vi "delete_document.vi"(11 "did":string) -> ()   [LabVIEW 2019]
panel:
  out "Device Out":T1
  in  "Device In":T1
  out "error out":errorcluster
  in  "error in":errorcluster
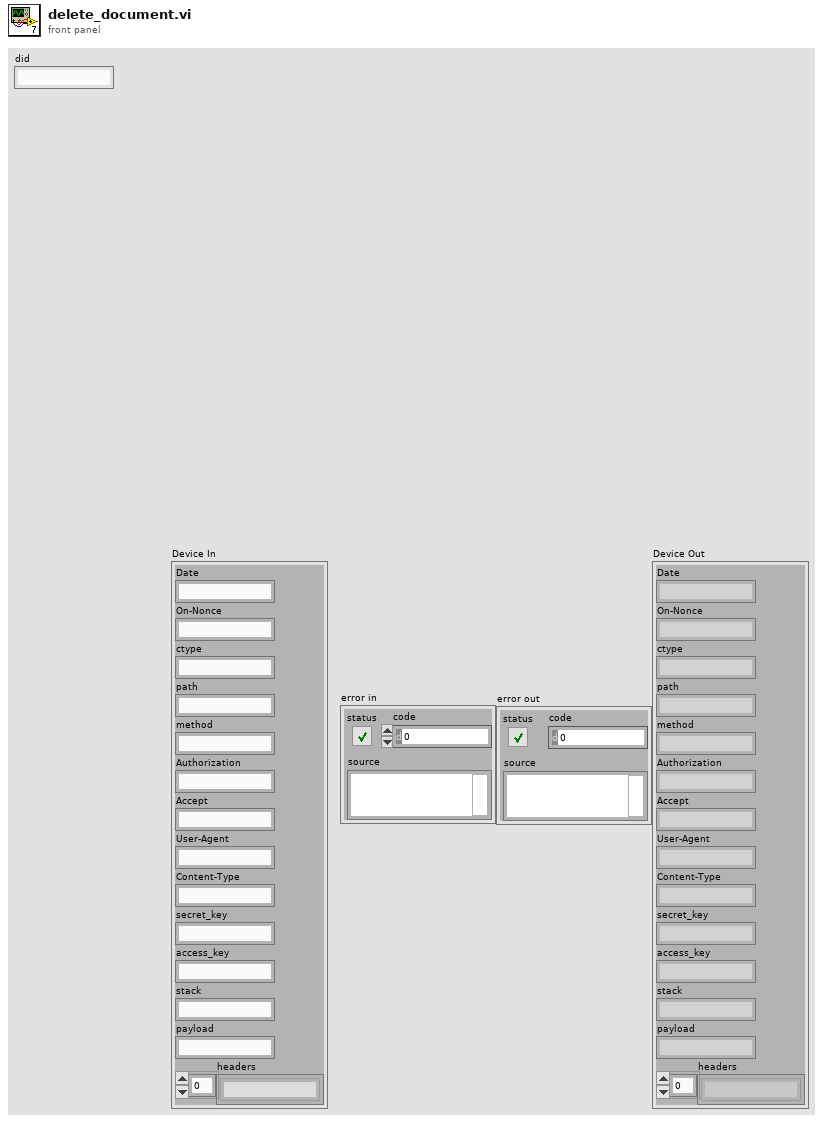
[diagram p1: front panel]
types:
  T1 = cluster{"Date":string, "On-Nonce":string, "ctype":string, "path":string, "method":string, "Authorization":string, "Accept":string, "User-Agent":string, "Content-Type":string, "secret_key":string, "access_key":string, "stack":string, "payload":string, "headers":string[]}
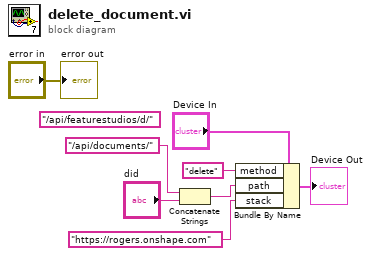
[diagram p0: block diagram]
diagram:
  (unwired) "/api/featurestudios/d/" ("payload")
  n1 = Concatenate Strings("/api/documents/" ("payload"), "did") -> (w2:string)
  n2 = Bundle By Name(cluster="Device In", "method"="delete" ("Method"), "path"=w2, "stack"="https://rogers.onshape.com" ("stacks")) -> (→"Device Out":T1)
  "error out" <- "error in"
